vi "Functions.vi"(8 "Error In":errorcluster, 10 "Function in":T1, 11 "Function ID in":u8) -> (0 "Error Out":errorcluster, 2 "Function ID out":u8, 3 "Function out":T1)   [LabVIEW 2011, in "Tinkerforge.lvlib" / "IP Connection.lvclass"]
doc: "This VI translates a function ID into a function enumeration and vice versa."
uses:
  IP Connection.lvclass
  Type Definitions/Functions.ctl
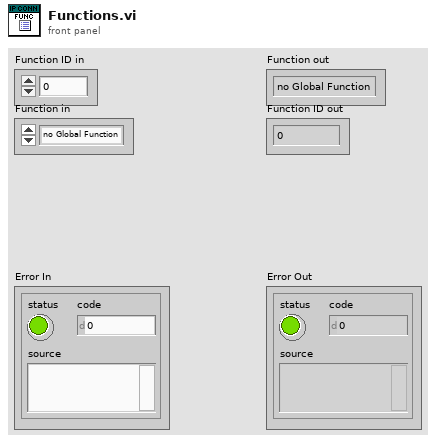
[diagram p1: front panel]
types:
  T1 = typedef "Tinkerforge.lvlib/IP Connection.lvclass/Functions.ctl" = enum8{"no Global Function", "get stack id", "enumerate", "CB enumerate"}
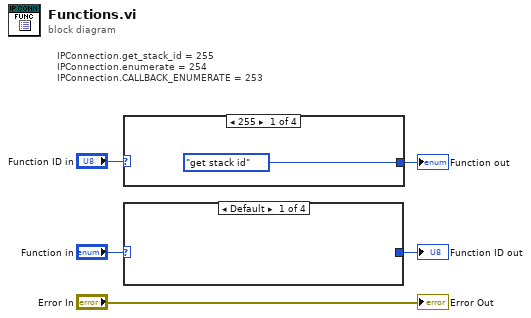
[diagram p0: block diagram]
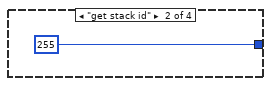
[diagram p2: hidden frame]
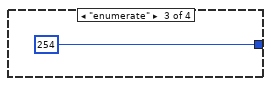
[diagram p3: hidden frame]
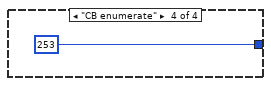
[diagram p4: hidden frame]
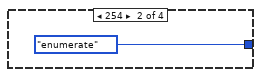
[diagram p5: hidden frame]
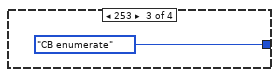
[diagram p6: hidden frame]
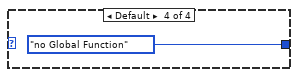
[diagram p7: hidden frame]
diagram:
  # "IPConnection.get_stack_id = 255\nIPConnection.enumerate = 254\nIPConnection.CALLBACK_ENUMERATE = 253"
  n1 = case shown="255" "Function ID in" {
    tunnel: [Functions."get stack id" ("Functions") Functions."enumerate" ("Functions") Functions."CB enumerate" ("Functions") Functions."no Global Function" ("Functions")] -> w3
    frame 255 {
    }
    frame 254 {
    }
    frame 253 {
    }
    frame Default {
    }
  }
  "Function out" <- w3
  n2 = case shown="Default" "Function in" {
    tunnel: [_ u8 255 u8 254 u8 253] -> w1
    frame Default {
    }
    frame "get stack id" {
    }
    frame "enumerate" {
    }
    frame "CB enumerate" {
    }
  }
  "Function ID out" <- w1
  "Error Out" <- "Error In"
